vi "XY Graph Compute Simple Plot Formula Event.vi"(8 "Error In":errorcluster, 11 "Mouse Click Event Data":T1) -> (0 "Error Out":errorcluster, 1 "Message":string, 2 "Formula":string, 3 "Plot Name":string, 5 "Graph Caption":string)   [LabVIEW 2021, in "XY Graph Add-Ons.lvlib"]
uses:
  XY Graph Add-Ons.lvlib
  XY Graph Mouse Click Event Data.ctl
  XY Graph Refnum.ctl
  <vilib>/Utility/miscctls.llb/LVPoint32TypeDef.ctl
  Get Plot at Mouse Click (XY Graph)/Get Plot at Mouse Click [AAC].vi
  XY Graph Add Single Plot with Name.vi
  Graphs.lvlib
  GUI/GUI.lvlib
  <vilib>/gmath/NI_Gmath.lvlib
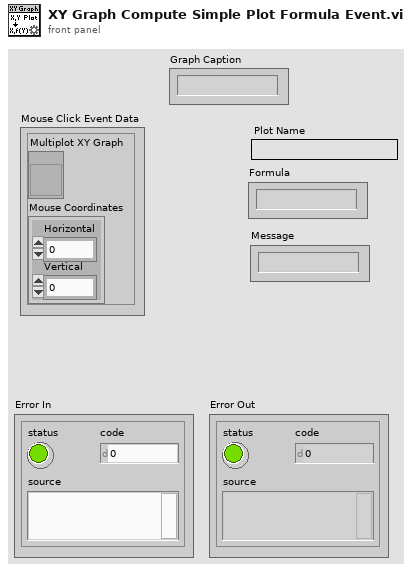
[diagram p1: front panel]
types:
  T1 = typedef "XY Graph Add-Ons.lvlib/XY Graph Mouse Click Event Data.ctl" = cluster{"Multiplot XY Graph":T2, "Mouse Coordinates":T3}
  T2 = typedef "XY Graph Add-Ons.lvlib/XY Graph Refnum.ctl" = refnum<vi>
  T3 = typedef "LVPoint32TypeDef.ctl" = cluster{"Horizontal":i32, "Vertical":i32}
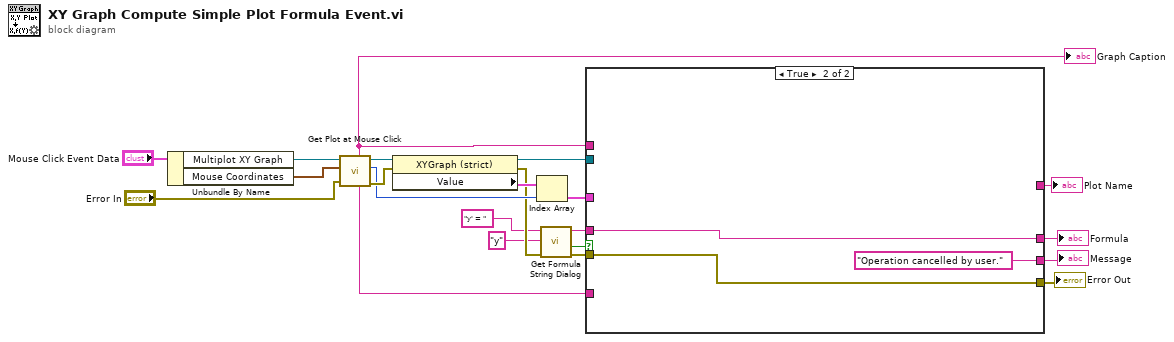
[diagram p0: block diagram]
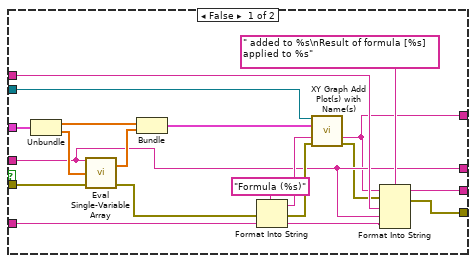
[diagram p2: hidden frame]
diagram:
  n1 = Unbundle By Name("Mouse Click Event Data") -> ("Multiplot XY Graph"=w21:T2, "Mouse Coordinates"=w20:T3)
  n2 = call-poly "Get Plot at Mouse Click.vi"("error in (no error)"="Error In", "Mouse Click Coordinates"=w20, "XYGraph Ref"=w21) -> ("error out"=w17:errorcluster, "Plot at Coordinates"=w15:i32, "XYGraph Ref"=w18:T2, "Plot Name"=w6:string, "Graph Name"=w5:string)  [unwired: 2 in, 2 out]
  "Graph Caption" <- w5
  n3 = property class="XYGraph (strict)"(reference=w18, error in=w17) -> (reference out=w9:T2, error out=w14:errorcluster, "Value"=w16:cluster{"X Array":dbl[], "Y Array":dbl[]}[])
  n4 = Index Array(array=w16, index=w15) -> (element=w13:cluster{"X Array":dbl[], "Y Array":dbl[]})
  n5 = call "Get Formula String Dialog.vi"("error in (no error)"=w14, "Variable (x)"="y", "Formula Name (f(x))"="y' = ") -> ("error out"=w12:errorcluster, "Cancelled?"=w7:bool, "Formula"=w11:string)  [unwired: 6 in]
  n6 = case shown="True" w7 {
    tunnel: w13 -> [w41 _]
    tunnel: w12 -> [w31 w44]
    tunnel: w11 -> [w27 w43]
    tunnel: [w27 w43] -> w10
    tunnel: w9 -> [w26 _]
    tunnel: [w23 w44] -> w8
    tunnel: w6 -> [w33 _]
    tunnel: w5 -> [w34 _]
    tunnel: [w32 "Operation cancelled by user."] -> w4
    tunnel: [w25 _] -> w3
    frame False {
      n7 = Unbundle(w41) -> ("X Array"=w40:dbl[], "Y Array"=w30:dbl[])
      n8 = call <vilib>:"Eval Single-Variable Array.vi"("error in (no error)"=w31, "X Values"=w30, "formula"=w27) -> ("error out"=w28:errorcluster, "Y Values"=w29:dbl[])
      n9 = Bundle("X Array"=w40, "Y Values"=w29) -> (w39:cluster{"X Array":dbl[], "Y Values":dbl[]})  [unwired: 1 in]
      n10 = Format Into String(format string="Formula (%s)" ("initial string"), error in=w28, w33) -> (resulting string=w38:string, error out=w37:errorcluster)  [unwired: 1 in]
      n11 = call-poly "XY Graph Add Plot(s) with Name(s).vi"("XYGraph Ref in"=w26, "Plot"=w39, "Plot Name (\"Plot\")"=w38, "error in (no error)"=w37) -> ("Plot Name"=w25:string, "error out"=w24:errorcluster)  [unwired: 8 in, 2 out]
      n12 = Format Into String(format string=" added to %s\nResult of formula [%s] applied to %s", initial string=w25, error in=w24, w34, w27, w33) -> (resulting string=w32:string, error out=w23:errorcluster)
    }
    frame True {
    }
  }
  "Error Out" <- w8
  "Formula" <- w10
  "Message" <- w4
  "Plot Name" <- w3
